vi "Setup UI.vi"(8 "error in (no error)":errorcluster, 10 "Set UI to input? (F)":bool, 11 "Analog Out Scan in":refnum<class "Analog Out Scan.lvclass">) -> (0 "error out":errorcluster, 3 "Analog Out Scan out":refnum<class "Analog Out Scan.lvclass">)   [LabVIEW 2017, in "Analog Out Scan.lvclass"]
doc: "Scanner::Setup is a constructor that has no parameters and faces the user. The Factory calls this VI to let the user configure this Scanner. It is dynamically dispatched in order to let the user choose the type as well as the options of the scanner."
uses:
  Analog Out Scan.lvclass
  Analog Out Scan.lvclass/Analog Out Scan.ctl
panel:
  in  "Channel":u8 max=1
  # "Analog Output Setup"
  # "No settable parameters yet"
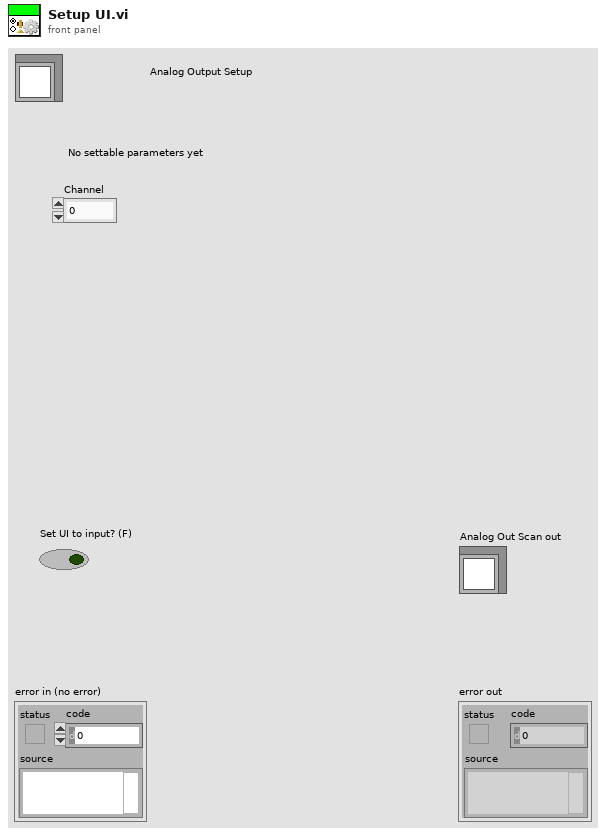
[diagram p1: front panel]
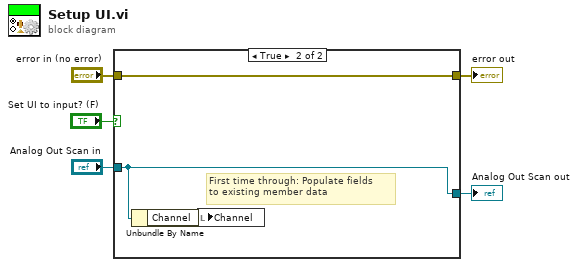
[diagram p0: block diagram]
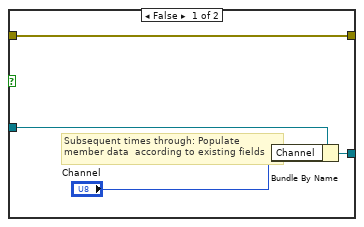
[diagram p2: hidden frame]
diagram:
  n1 = case shown="True" "Set UI to input? (F)" {
    tunnel: [w8 w12] -> w3
    tunnel: "Analog Out Scan in" -> [w9 w12]
    tunnel: "error in (no error)" -> [w6 w10]
    tunnel: [w6 w10] -> w1
    frame False {
      # "Subsequent times through: Populate \nmember data  according to existing fields"
      n2 = Bundle By Name(cluster=w9, "Channel"="Channel") -> (w8:refnum<class "Analog Out Scan.lvclass">)
    }
    frame True {
      # "First time through: Populate fields  \nto existing member data"
      n3 = Unbundle By Name(w12) -> ("Channel"=w11:u8)
      n4 = local write "Channel"(w11) -> ()
    }
  }
  "error out" <- w1
  "Analog Out Scan out" <- w3
